vi "Max Read Single.vi"(8 "error in":errorcluster, 9 "Channel Index":i32=1, 11 "Max Voltage Limit in":refnum<class "Voltage Limit.lvclass">) -> (0 "error out":errorcluster, 1 "Changed or First Call?":bool, 2 "Voltage Max SP":dbl, 3 "Max Voltage Limit out":refnum<class "Voltage Limit.lvclass">)   [LabVIEW 2023, in "Voltage Limit.lvclass"]
uses:
  Voltage Limit.lvclass
  Parents/Limit/Limit.lvclass
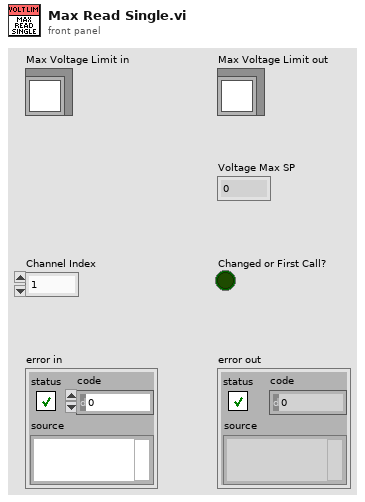
[diagram p1: front panel]
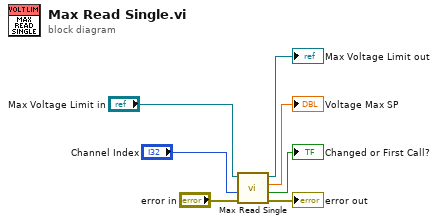
[diagram p0: block diagram]
diagram:
  n1 = call-parent "Max Read Single.vi"("error in"="error in", "Channel Index"="Channel Index", "Max Limit in"="Max Voltage Limit in") -> ("error out"=→"error out":errorcluster, "Changed or First Call?"=→"Changed or First Call?":bool, "Current Max SP"=→"Voltage Max SP":dbl, "Max Limit out"=→"Max Voltage Limit out":refnum<class "Voltage Limit.lvclass">)  [unwired: 5 in]
